vi "Get DDGIOC Trigger.vi"(11 "trigger":u32) -> (2 "function return":u32, 3 "trigger out":u32)   [LabVIEW 2018, in "Copy of Andor SDK.lvlib"]
doc: "EXPNETTYPE unsigned int WINAPI GetDDGIOCTrigger(at_u32 * trigger);"
uses:
  Copy of Andor SDK.lvlib
  <userlib>/Andor SDK/ATMCD32D.dll
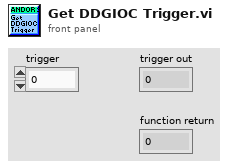
[diagram p1: front panel]
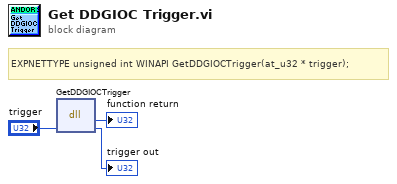
[diagram p0: block diagram]
diagram:
  # "EXPNETTYPE unsigned int WINAPI GetDDGIOCTrigger(at_u32 * trigger);"
  n1 = dll-call lib="C:/Program Files (x86)/National Instruments/LabVIEW 2018/user.lib/Andor SDK/ATMCD32D.*" fn="GetDDGIOCTrigger"("trigger"="trigger") -> (→"function return":u32, "trigger"=→"trigger out":u32)  [unwired: 3 in, 2 out]
